vi "NiXnet CreateSession.vi"(6 "contextId":T1, 8 "error in":errorcluster, 9 "timeout (ms)":i32=-1, 10 "Request Data":T4, 11 "gRPC ID":T1) -> (0 "error out":errorcluster, 2 "Response Data":T2, 3 "gRPC ID out":T1)   [LabVIEW 2024, in "grpc-xnet_client.lvlib"]
uses:
  grpc-xnet_client.lvlib
  RPC Messages/nixnet_grpc_CreateSessionRequest_mode_enum/nixnet_grpc_CreateSessionRequest_mode_enum.lvclass
  RPC Messages/nixnet_grpc_CreateSessionRequest_mode_enum/nixnet_grpc_CreateSessionRequest_mode_enum.lvclass/nixnet_grpc_CreateSessionRequest_mode_enum.ctl
  14035477-4c25-4107-8ed5-d0c4ef420ce5.vi
  RPC Messages/nidevice_grpc_Session_Flat.ctl
  RPC Messages/nixnet_grpc_CreateSessionResponse_Flat.ctl
  <vilib>/gRPC/LabVIEW gRPC Library/Shared/grpcId.ctl
  <vilib>/gRPC/LabVIEW gRPC Library/grpc-lvsupport-release.lvlib
  RPC Messages/nidevice_grpc_Session.ctl
  RPC Messages/nixnet_grpc_CreateSessionResponse.ctl
  RPC Messages/nidevice_grpc_SessionInitializationBehavior.ctl
  RPC Messages/nixnet_grpc_CreateSessionRequest.ctl
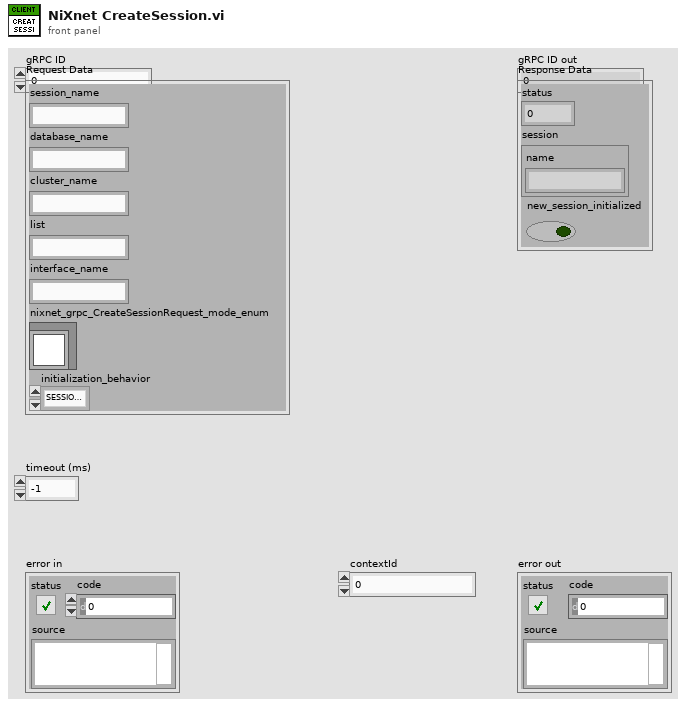
[diagram p1: front panel]
types:
  T1 = typedef "grpc-lvsupport-release.lvlib/grpcId.ctl" = u64
  T2 = typedef "grpc-xnet_client.lvlib/nixnet_grpc_CreateSessionResponse.ctl" = cluster{"status":i32, "session":T3, "new_session_initialized":bool}
  T3 = typedef "grpc-xnet_client.lvlib/nidevice_grpc_Session.ctl" = cluster{"name":string}
  T4 = typedef "grpc-xnet_client.lvlib/nixnet_grpc_CreateSessionRequest.ctl" = cluster{"session_name":string, "database_name":string, "cluster_name":string, "list":string, "interface_name":string, "nixnet_grpc_CreateSessionRequest_mode_enum":refnum<class "nixnet_grpc_CreateSessionRequest_mode_enum.lvclass">, "initialization_behavior":T5}
  T5 = typedef "grpc-xnet_client.lvlib/nidevice_grpc_SessionInitializationBehavior.ctl" = enum32{"SESSION_INITIALIZATION_BEHAVIOR_UNSPECIFIED", "SESSION_INITIALIZATION_BEHAVIOR_INITIALIZE_NEW", "SESSION_INITIALIZATION_BEHAVIOR_ATTACH_TO_EXISTING"}
  T6 = typedef "grpc-xnet_client.lvlib/nixnet_grpc_CreateSessionResponse_Flat.ctl" = cluster{"status":i32, "session":T7, "new_session_initialized":bool}
  T7 = typedef "grpc-xnet_client.lvlib/nidevice_grpc_Session_Flat.ctl" = cluster{"name":string}
  T8 = typedef "grpc-xnet_client.lvlib/nixnet_grpc_CreateSessionRequest_Flat.ctl" = cluster{"session_name":string, "database_name":string, "cluster_name":string, "list":string, "interface_name":string, "nixnet_grpc_CreateSessionRequest_mode_enum_selected_index":i32, "mode":T9, "mode_raw":u32, "initialization_behavior":T5}
  T9 = typedef "grpc-xnet_client.lvlib/nixnet_grpc_CreateSessionMode.ctl" = enum32{"CREATE_SESSION_MODE_SIGNAL_IN_SINGLE_POINT", "CREATE_SESSION_MODE_SIGNAL_IN_WAVEFORM", "CREATE_SESSION_MODE_SIGNAL_IN_XY", "CREATE_SESSION_MODE_SIGNAL_OUT_SINGLE_POINT", "CREATE_SESSION_MODE_SIGNAL_OUT_WAVEFORM", "CREATE_SESSION_MODE_SIGNAL_OUT_XY", "CREATE_SESSION_MODE_FRAME_IN_STREAM", "CREATE_SESSION_MODE_FRAME_IN_QUEUED", "CREATE_SESSION_MODE_FRAME_IN_SINGLE_POINT", "CREATE_SESSION_MODE_FRAME_OUT_STREAM", "CREATE_SESSION_MODE_FRAME_OUT_QUEUED", "CREATE_SESSION_MODE_FRAME_OUT_SINGLE_POINT", "CREATE_SESSION_MODE_SIGNAL_CONVERSION_SINGLE_POINT"}
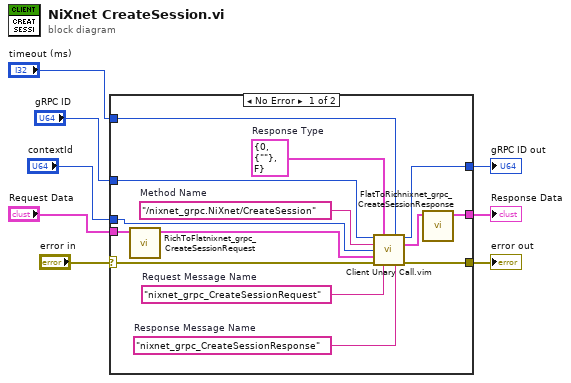
[diagram p0: block diagram]
diagram:
  n1 = case shown="No Error" "error in" {
    selector: "error in" -> [w18 w23]
    tunnel: [w17 w23] -> w7
    tunnel: "gRPC ID" -> [w16 w24]
    tunnel: [w15 w24] -> w5
    tunnel: "Request Data" -> [w12 _]
    tunnel: [w9 _] -> w3
    tunnel: "timeout (ms)" -> [w14 _]
    tunnel: "contextId" -> [w13 _]
    frame No Error {
      w19 = "nixnet_grpc_CreateSessionResponse"  # Response Message Name
      w20 = "nixnet_grpc_CreateSessionRequest"  # Request Message Name
      w21 = T6 {"status"=0, "session"={"name"=""}, "new_session_initialized"=FALSE}  # Response Type
      w22 = "/nixnet_grpc.NiXnet/CreateSession"  # Method Name
      n2 = call "RichToFlatnixnet_grpc_CreateSessionRequest.vi"("InputCluster"=w12) -> ("OutputCluster"=w11:T8)  [unwired: 10 in]
      n3 = call "Client Unary Call.vim"("ClientID in"=w16, "Response Type"=w21, "timeout (ms)"=w14, "Method Name"=w22, "contextId"=w13, "Request Data"=w11, "error in"=w18, "Request Message Name"=w20, "Response Message Name"=w19) -> ("ClientID out"=w15:u64, "Response Data"=w10:T6, "error out"=w17:errorcluster)  [unwired: 4 in]
      n4 = call "FlatToRichnixnet_grpc_CreateSessionResponse.vi"("InputCluster"=w10) -> ("OutputCluster"=w9:T2)  [unwired: 10 in]
    }
    frame Error {
    }
  }
  "error out" <- w7
  "gRPC ID out" <- w5
  "Response Data" <- w3
